vi "Reset Encoder_X.vi"   [LabVIEW 2010, in "4134Outputs.lvlib"]
uses:
  4134Outputs.lvlib
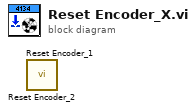
[diagram p0: block diagram]
diagram:
  n1 = call "Reset Encoder_2.vi"() -> ()  [unwired: 10 in, 1 out]
  n2 = call "Reset Encoder_1.vi"() -> ()  [unwired: 10 in, 1 out]
